vi "Get Version.vi"(8 "error in (no error)":errorcluster, 11 "UDPlog Configurations in":refnum<class "UDPlog Configurations.lvclass">) -> (0 "error out":errorcluster, 2 "version":T1, 3 "UDPlog Configurations out":refnum<class "UDPlog Configurations.lvclass">)   [LabVIEW 2023, in "UDPlog.lvlib" / "UDPlog Configurations.lvclass"]
uses:
  UDPlog Configurations.lvclass
  Users/Public/Documents/National Instruments/NI VeriStand 2023/Custom Devices/Data Sharing Framework/Linux_x64/DSF Core.lvlibp/Typedefs/DSF Version Info.ctl
  Users/Public/Documents/National Instruments/NI VeriStand 2023/Custom Devices/Data Sharing Framework/Linux_x64/DSF Core.lvlibp
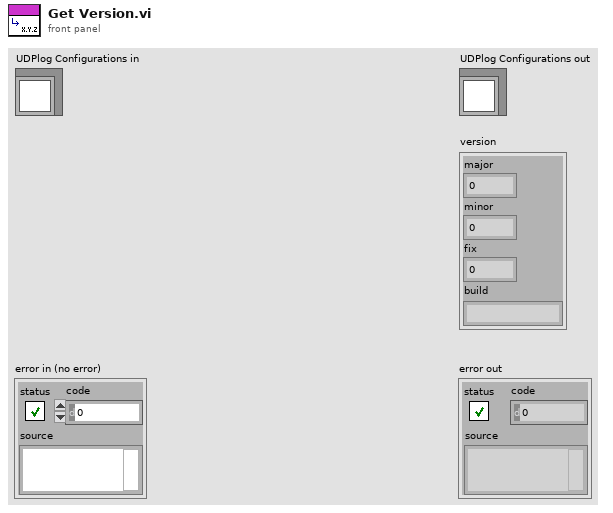
[diagram p1: front panel]
types:
  T1 = typedef "DSF Core.lvlibp/DSF Version Info.ctl" = cluster{"major":u32, "minor":u32, "fix":u32, "build":string}
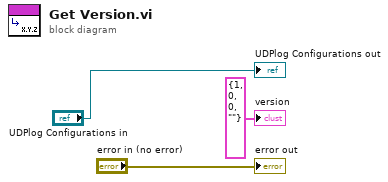
[diagram p0: block diagram]
diagram:
  "error out" <- "error in (no error)"
  "UDPlog Configurations out" <- "UDPlog Configurations in"
  "version" <- T1 {"major"=1, "minor"=0, "fix"=0, "build"=""} ("version")
